vi "People Tracking Globals.vi"() -> ()   [LabVIEW 2014]
panel:
  in  "Size Gain":dbl=1e-05
  in  "Heading Gain":dbl=0.8
  in  "Luma Range":cluster{"Lower value":i32, "Upper value":i32}={"Lower value"=3, "Upper value"=80}
  in  "Sat Range":cluster{"Lower value":i32, "Upper value":i32}={"Lower value"=205, "Upper value"=250}
  in  "Hue Range":cluster{"Lower value":i32, "Upper value":i32}={"Lower value"=237, "Upper value"=255}
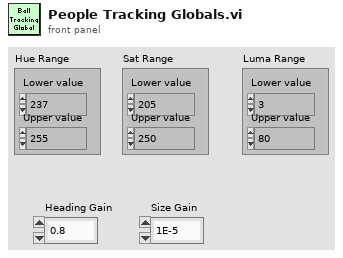
[diagram p1: front panel]
diagram:
